vi "bh3_lifesign.vi"(8 "error in (no error)":errorcluster, 11 "bt connection ID in":refnum<k31>) -> (0 "error out":errorcluster, 3 "bt connection ID out":refnum<k31>)   [LabVIEW 2013]
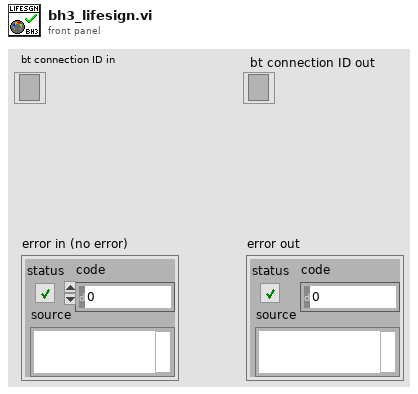
[diagram p1: front panel]
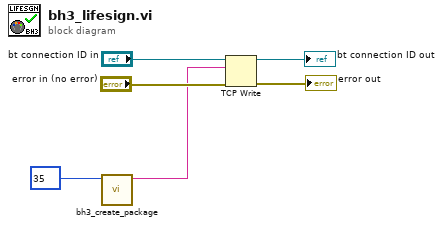
[diagram p0: block diagram]
diagram:
  n1 = call "bh3_create_package.vi"("msg_ID"=u8 35) -> ("package string"=w3:string)  [unwired: 9 in, 1 out]
  n2 = TCP Write(connection ID="bt connection ID in", data in=w3, error in (no error)="error in (no error)") -> (connection ID out=→"bt connection ID out":refnum<k31>, error out=→"error out":errorcluster)  [unwired: 1 in, 1 out]
